vi "AFS Calculatte DCAP_Percentage.vi"(6 "Data2 In":string[](array[string]), 8 "Error In":errorcluster, 9 "Target Cap (fF)":dbl, 11 "Data1 In":string[](array[string])) -> (0 "Error Out":errorcluster, 3 "Delta C":string[](array[string]), 4 "% Detla C":string[](array[string]))   [LabVIEW 2017]
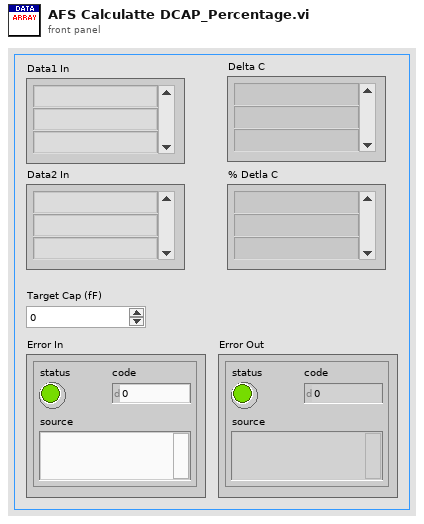
[diagram p1: front panel]
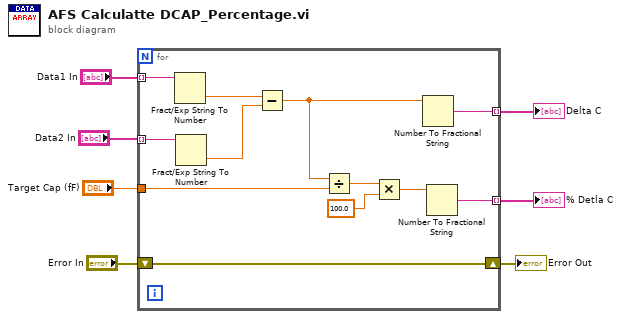
[diagram p0: block diagram]
diagram:
  n1 = for {
    tunnel: "Data1 In" -> [w19] mode=indexing
    tunnel: "Data2 In" -> [w17] mode=indexing
    tunnel: [w14] -> w3 mode=indexing
    tunnel: "Target Cap (fF)" -> [w13]
    tunnel: [w12] -> w4 mode=indexing
    shift-right: [w8] -> w1
    shift-left: "Error In" -> [w8]
    n2 = Fract/Exp String To Number(string=w19) -> (number=w18:dbl)  [unwired: 3 in, 1 out]
    n3 = Fract/Exp String To Number(string=w17) -> (number=w16:dbl)  [unwired: 3 in, 1 out]
    n4 = Subtract(x=w18, y=w16) -> (x-y=w15:dbl)
    n5 = Divide(x=w15, y=w13) -> (x/y=w10:dbl)
    n6 = Multiply(x=w10, y=100.0) -> (x*y=w11:dbl)
    n7 = Number To Fractional String(number=w15) -> (F-format string=w14:string)  [unwired: 3 in]
    n8 = Number To Fractional String(number=w11) -> (F-format string=w12:string)  [unwired: 3 in]
  }
  "Error Out" <- w1
  "Delta C" <- w3
  "% Detla C" <- w4
